vi "Read Base path.vi"(8 "error in (no error)":errorcluster, 11 "CV-Storage in":refnum<class "CV-Storage.lvclass">) -> (0 "error out":errorcluster, 2 "Base path":path, 3 "CV-Storage out":refnum<class "CV-Storage.lvclass">)   [LabVIEW 2013, in "CameraVision.lvlib" / "CV-Storage.lvclass"]
uses:
  CV-Storage.lvclass
  CV-Storage.lvclass/CV-Storage.ctl
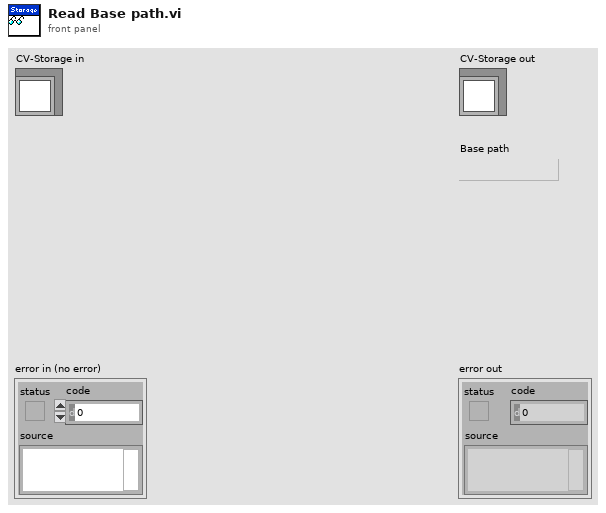
[diagram p1: front panel]
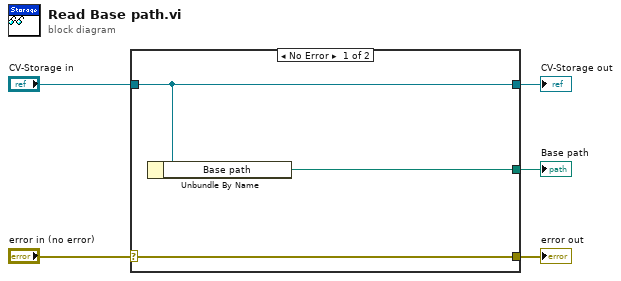
[diagram p0: block diagram]
diagram:
  n1 = case shown="No Error" "error in (no error)" {
    selector: "error in (no error)" -> [w8 w9]
    tunnel: [w8 w9] -> w4
    tunnel: [w7 w10] -> w2
    tunnel: "CV-Storage in" -> [w7 w10]
    tunnel: [w6 _] -> w1
    frame No Error {
      n2 = Unbundle By Name(w7) -> ("Base path"=w6:path)
    }
    frame Error {
    }
  }
  "error out" <- w4
  "CV-Storage out" <- w2
  "Base path" <- w1
